vi "Release.vi"(8 "error in (no error)":errorcluster, 11 "VacuumLines in":refnum<class "VacuumLines.lvclass">) -> (0 "error out":errorcluster, 3 "VacuumLines out":refnum<class "VacuumLines.lvclass">)   [LabVIEW 2016, in "Hardware.lvlib" / "VacuumLine.lvlib" / "VacuumLines.lvclass"]
uses:
  <userlib>/Common Components/Hardware/Abstract System/VacuumLine/VacuumLines/VacuumLines.lvclass
  <userlib>/Common Components/Hardware/Abstract System/VacuumLine/VacuumLines/VacuumLines.lvclass/VacuumLines.ctl
  <userlib>/Common Components/Hardware/Thermometer/Thermometer.lvclass
  <userlib>/Common Components/Hardware/GaugeController/GaugeController/GaugeController.lvclass
  <userlib>/Common Components/Hardware/Abstract System/VacuumLine/VacuumLine/VacuumLine.lvclass
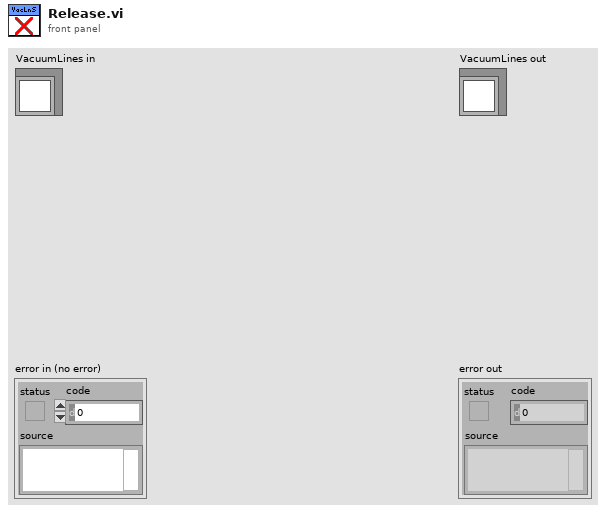
[diagram p1: front panel]
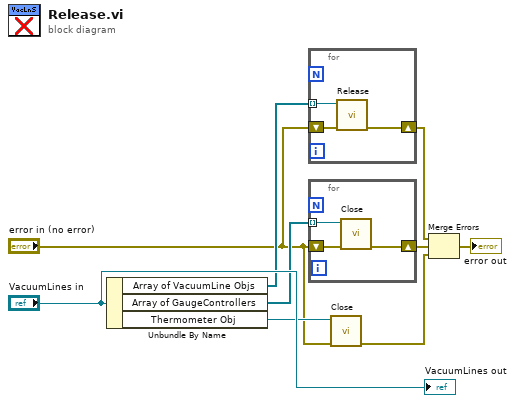
[diagram p0: block diagram]
diagram:
  n1 = Unbundle By Name("VacuumLines in") -> ("Array of VacuumLine Objs"=w8:refnum<class "VacuumLine.lvclass">[], "Array of GaugeControllers"=w6:refnum<class "GaugeController.lvclass">[], "Thermometer Obj"=w3:refnum<class "Thermometer.lvclass">)
  n2 = for {
    tunnel: w8 -> [w12] mode=indexing
    shift-right: [w10] -> w7
    shift-left: "error in (no error)" -> [w11]
    n3 = call <userlib>:"Release.vi"("error in (no error)"=w11, "VacuumLine in"=w12) -> ("error out"=w10:errorcluster)  [unwired: 8 in, 1 out]
  }
  n4 = for {
    tunnel: w6 -> [w15] mode=indexing
    shift-right: [w13] -> w4
    shift-left: "error in (no error)" -> [w14]
    n5 = call-dynamic "Close.vi"("error in (no error)"=w14, "GaugeController in"=w15) -> ("error out"=w13:errorcluster)  [unwired: 8 in, 1 out]
  }
  n6 = call-dynamic "Close.vi"("error in (no error)"="error in (no error)", "Thermometer in"=w3) -> ("error out"=w1:errorcluster)  [unwired: 8 in, 1 out]
  n7 = Merge Errors(w7, w4, w1) -> (→"error out":errorcluster)
  "VacuumLines out" <- "VacuumLines in"
